vi "Initialize Controls and Indicators.vi"(7 "Set min panel sizes?":bool=TRUE, 8 "error in (no error)":errorcluster, 11 "VI in":refnum<vi>) -> (0 "error out":errorcluster)   [LabVIEW 2020, in "Execution UI V2.lvclass"]
uses:
  Execution UI V2.lvclass
  TypeDefs/Color Theme.ctl
  <vilib>/Utility/miscctls.llb/LVPointTypeDef.ctl
  Execution UI V2.lvclass/Execution UI V2.ctl
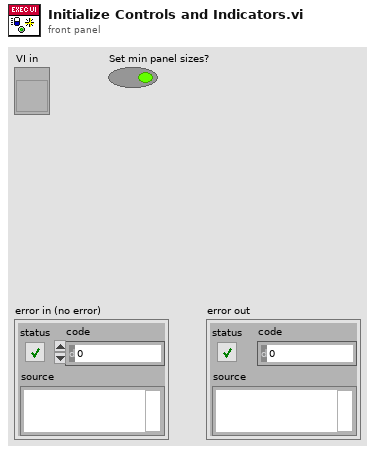
[diagram p1: front panel]
types:
  T1 = typedef "Execution UI V2.lvclass/Color Theme.ctl" = cluster{"Primary":u32, "Primary Light":u32, "Primary Dark":u32, "Accent":u32, "Primary Text":u32, "Secondary Text":u32}
  T2 = typedef "LVPointTypeDef.ctl" = cluster{"Horizontal":i16, "Vertical":i16}
  T3 = enum8{"Enabled", "Disabled", "Disabled and Grayed Out"}
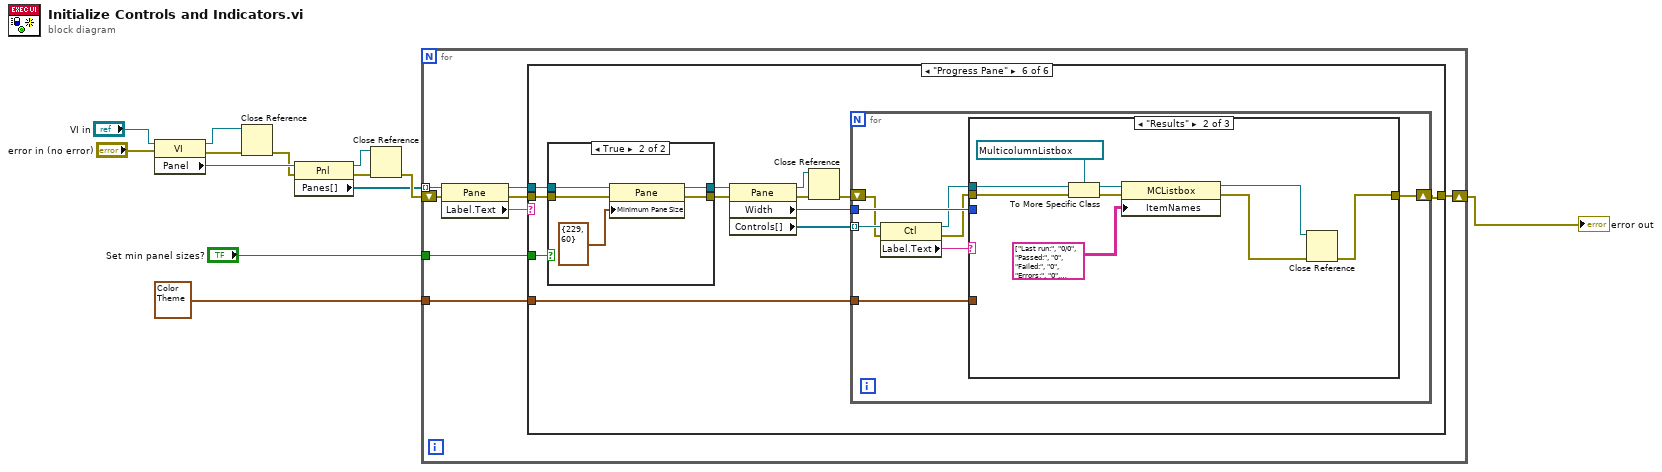
[diagram p0: block diagram]
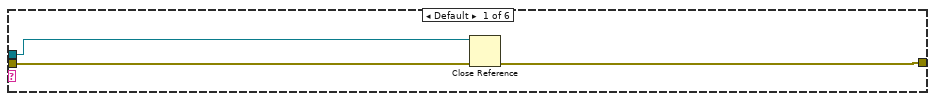
[diagram p2: hidden frame]
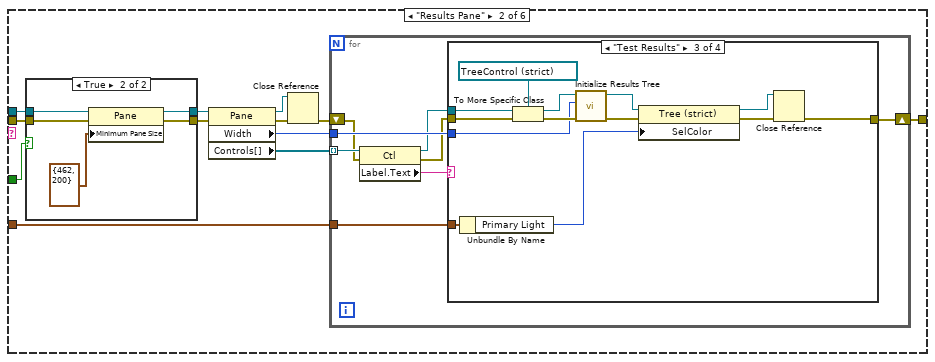
[diagram p3: hidden frame]
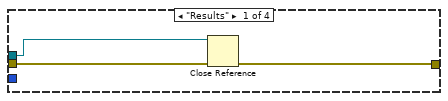
[diagram p5: hidden frame]
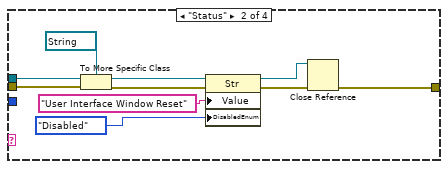
[diagram p6: hidden frame]
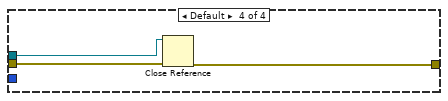
[diagram p7: hidden frame]
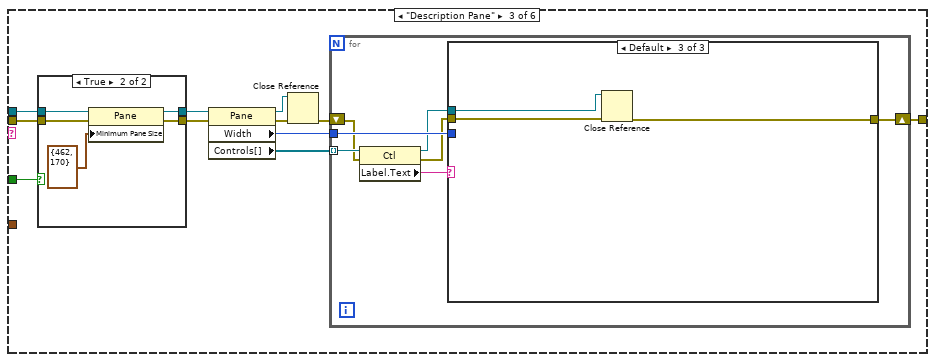
[diagram p8: hidden frame]
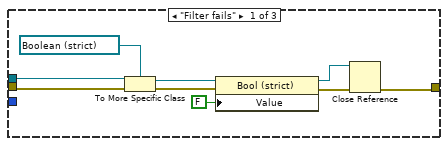
[diagram p10: hidden frame]
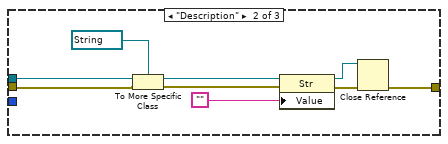
[diagram p11: hidden frame]
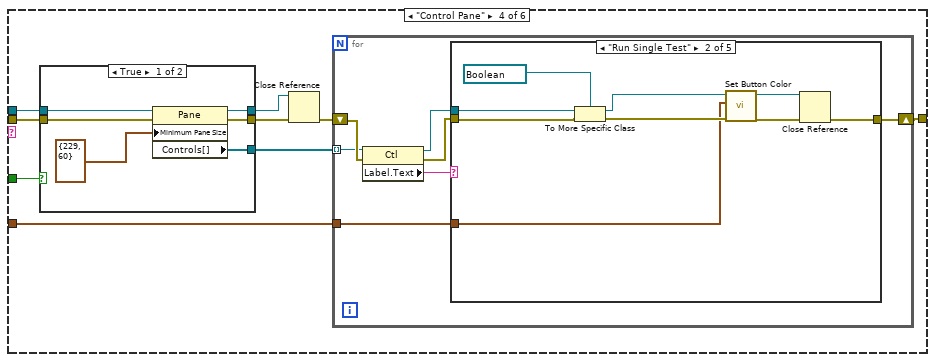
[diagram p12: hidden frame]
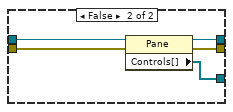
[diagram p13: hidden frame]
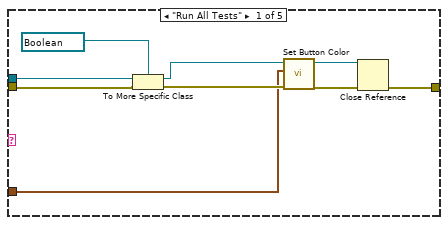
[diagram p14: hidden frame]
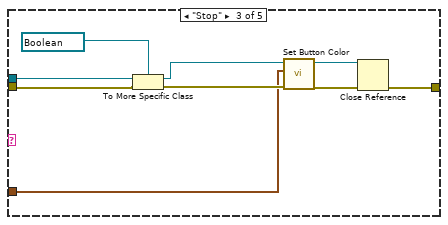
[diagram p15: hidden frame]
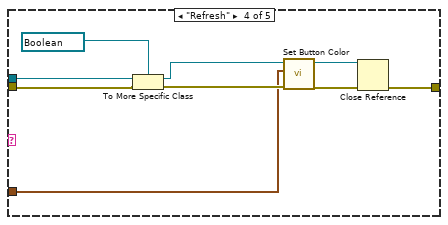
[diagram p16: hidden frame]
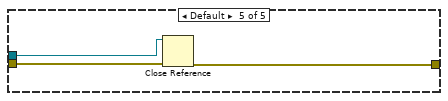
[diagram p17: hidden frame]
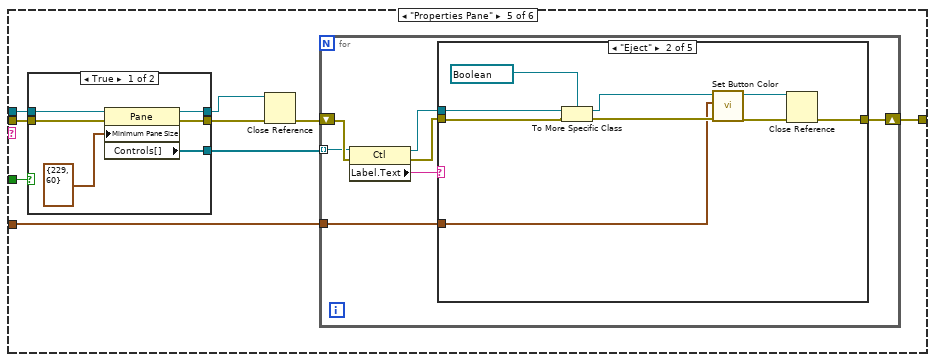
[diagram p18: hidden frame]
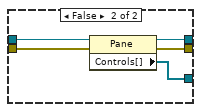
[diagram p19: hidden frame]
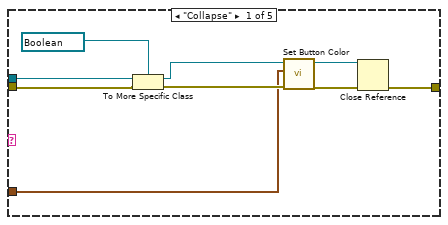
[diagram p20: hidden frame]
diagram:
  n1 = property class="VI"(reference="VI in", error in="error in (no error)") -> (reference out=w3:refnum<vi>, error out=w5:errorcluster, "Panel"=w12:refnum<vi>)
  n2 = Close Reference(reference=w3, error in (no error)=w5) -> (error out=w4:errorcluster)
  n3 = property class="Pnl"(reference=w12, error in=w4) -> (reference out=w8:refnum<vi>, error out=w7:errorcluster, "Panes[]"=w6:refnum<vi>[])
  n4 = Close Reference(reference=w8, error in (no error)=w7) -> (error out=w9:errorcluster)
  n5 = for {
    tunnel: w6 -> [w21] mode=indexing
    shift-right: [w18] -> w10
    shift-left: w9 -> [w17]
    tunnel: T1 {"Primary"=6323595, "Primary Light"=13621468, "Primary Dark"=4545124, "Accent"=10395294, "Primary Text"=2171169, "Secondary Text"=7697781} ("Color Theme") -> [w15]
    tunnel: "Set min panel sizes?" -> [w14]
    n6 = property class="Pane"(reference=w21, error in=w17) -> (reference out=w19:refnum<vi>, error out=w16:errorcluster, "Label.Text"=w20:string)
    n7 = case shown="\"Progress Pane\"" w20 {
      tunnel: w19 -> [w22 w29 w84 w135 w201 w262]
      tunnel: [w23 w34 w89 w130 w196 w261] -> w18
      tunnel: w16 -> [w24 w27 w82 w134 w200 w263]
      tunnel: w15 -> [_ w26 _ w129 w194 w260]
      tunnel: w14 -> [_ w25 w81 w127 w193 w259]
      frame Default {
        n8 = Close Reference(reference=w22, error in (no error)=w24) -> (error out=w23:errorcluster)
      }
      frame "Results Pane" {
        n9 = case shown="True" w25 {
          tunnel: [w38 w43] -> w30
          tunnel: w29 -> [w38 w42]
          tunnel: [w37 w41] -> w28
          tunnel: w27 -> [w37 w40]
          frame False {
          }
          frame True {
            n10 = property class="Pane"(reference=w42, error in=w40, "Minimum Pane Size"=T2 {"Horizontal"=462, "Vertical"=200}) -> (reference out=w43:refnum<vi>, error out=w41:errorcluster)
          }
        }
        n11 = property class="Pane"(reference=w30, error in=w28) -> (reference out=w31:refnum<vi>, error out=w33:errorcluster, "Width"=w36:u32, "Controls[]"=w35:refnum<vi>[])
        n12 = Close Reference(reference=w31, error in (no error)=w33) -> (error out=w32:errorcluster)
        n13 = for {
          tunnel: w36 -> [w51]
          tunnel: w35 -> [w50] mode=indexing
          shift-right: [w45] -> w34
          shift-left: w32 -> [w46]
          tunnel: w26 -> [w44]
          n14 = property class="Ctl"(reference=w50, error in=w46) -> (reference out=w48:refnum<vi>, error out=w47:errorcluster, "Label.Text"=w49:string)
          n15 = case shown="\"Test Results\"" w49 {
            tunnel: w51 -> [_ _ w72 _]
            tunnel: w48 -> [w52 w63 w76 w78]
            tunnel: w47 -> [w54 w62 w77 w80]
            tunnel: [w53 w56 w68 w79] -> w45
            tunnel: w44 -> [_ _ w66 _]
            frame "Results" {
              n16 = Close Reference(reference=w52, error in (no error)=w54) -> (error out=w53:errorcluster)
            }
            frame "Status" {
              n17 = To More Specific Class(target class=refnum<vi> refnum ("reference"), reference=w63, error in=w62) -> (specific class reference=w61:refnum<vi>, error out=w60:errorcluster)
              n18 = property on="Property Node" class="Str"(reference=w61, error in=w60, "Value"="User Interface Window Reset" ("Item Names"), "DisabledEnum"=T3."Disabled" ("Disabled")) -> (reference out=w57:refnum<vi>, error out=w58:errorcluster)
              n19 = Close Reference(reference=w57, error in (no error)=w58) -> (error out=w56:errorcluster)
            }
            frame "Test Results" {
              n20 = Unbundle By Name(w66) -> ("Primary Light"=w65:u32)
              n21 = To More Specific Class(target class=refnum<vi> refnum ("reference"), reference=w76, error in=w77) -> (specific class reference=w74:refnum<vi>, error out=w75:errorcluster)
              n22 = call "Initialize Results Tree.vi"("error in (no error)"=w75, "Pane width"=w72, "TreeControl in"=w74) -> ("error out"=w70:errorcluster, "reference out"=w71:refnum<vi>)  [unwired: 7 in]
              n23 = property class="Tree (strict)"(reference=w71, error in=w70, "SelColor"=w65) -> (reference out=w67:refnum<vi>, error out=w69:errorcluster)
              n24 = Close Reference(reference=w67, error in (no error)=w69) -> (error out=w68:errorcluster)
            }
            frame Default {
              n25 = Close Reference(reference=w78, error in (no error)=w80) -> (error out=w79:errorcluster)
            }
          }
        }
      }
      frame "Description Pane" {
        n26 = case shown="True" w81 {
          tunnel: [w93 w98] -> w85
          tunnel: w84 -> [w93 w97]
          tunnel: [w92 w96] -> w83
          tunnel: w82 -> [w92 w95]
          frame False {
          }
          frame True {
            n27 = property class="Pane"(reference=w97, error in=w95, "Minimum Pane Size"=T2 {"Horizontal"=462, "Vertical"=170}) -> (reference out=w98:refnum<vi>, error out=w96:errorcluster)
          }
        }
        n28 = property class="Pane"(reference=w85, error in=w83) -> (reference out=w86:refnum<vi>, error out=w88:errorcluster, "Width"=w91:u32, "Controls[]"=w90:refnum<vi>[])
        n29 = Close Reference(reference=w86, error in (no error)=w88) -> (error out=w87:errorcluster)
        n30 = for {
          tunnel: w91 -> [w105]
          tunnel: w90 -> [w104] mode=indexing
          shift-right: [w99] -> w89
          shift-left: w87 -> [w100]
          n31 = property class="Ctl"(reference=w104, error in=w100) -> (reference out=w102:refnum<vi>, error out=w101:errorcluster, "Label.Text"=w103:string)
          n32 = case shown="Default" w103 {
            tunnel: w105 -> [_ _ _]
            tunnel: w102 -> [w108 w123 w124]
            tunnel: w101 -> [w109 w118 w126]
            tunnel: [w110 w120 w125] -> w99
            frame "Filter fails" {
              n33 = To More Specific Class(target class=refnum<vi> refnum ("Filter fails"), reference=w108, error in=w109) -> (specific class reference=w112:refnum<vi>, error out=w111:errorcluster)
              n34 = property on="Property Node" class="Bool (strict)"(reference=w112, error in=w111, "Value"=FALSE) -> (reference out=w113:refnum<vi>, error out=w114:errorcluster)
              n35 = Close Reference(reference=w113, error in (no error)=w114) -> (error out=w110:errorcluster)
            }
            frame "Description" {
              n36 = To More Specific Class(target class=refnum<vi> refnum ("reference"), reference=w123, error in=w118) -> (specific class reference=w119:refnum<vi>, error out=w117:errorcluster)
              n37 = property on="Property Node" class="Str"(reference=w119, error in=w117, "Value"="") -> (reference out=w121:refnum<vi>, error out=w122:errorcluster)
              n38 = Close Reference(reference=w121, error in (no error)=w122) -> (error out=w120:errorcluster)
            }
            frame Default {
              n39 = Close Reference(reference=w124, error in (no error)=w126) -> (error out=w125:errorcluster)
            }
          }
        }
      }
      frame "Control Pane" {
        n40 = case shown="True" w127 {
          tunnel: w135 -> [w140 w146]
          tunnel: w134 -> [w139 w145]
          tunnel: [w138 w144] -> w133
          tunnel: [w137 w143] -> w132
          tunnel: [w136 w142] -> w128
          frame True {
            n41 = property class="Pane"(reference=w140, error in=w139, "Minimum Pane Size"=T2 {"Horizontal"=229, "Vertical"=60}) -> (reference out=w137:refnum<vi>, error out=w138:errorcluster, "Controls[]"=w136:refnum<vi>[])
          }
          frame False {
            n42 = property class="Pane"(reference=w146, error in=w145) -> (reference out=w143:refnum<vi>, error out=w144:errorcluster, "Controls[]"=w142:refnum<vi>[])
          }
        }
        n43 = Close Reference(reference=w132, error in (no error)=w133) -> (error out=w131:errorcluster)
        n44 = for {
          shift-right: [w149] -> w130
          shift-left: w131 -> [w150]
          tunnel: w129 -> [w148]
          tunnel: w128 -> [w147] mode=indexing
          n45 = property class="Ctl"(reference=w147, error in=w150) -> (reference out=w152:refnum<vi>, error out=w151:errorcluster, "Label.Text"=w153:string)
          n46 = case shown="\"Run Single Test\"" w153 {
            tunnel: w152 -> [w162 w171 w180 w189 w190]
            tunnel: w151 -> [w160 w169 w178 w187 w192]
            tunnel: [w161 w170 w179 w188 w191] -> w149
            tunnel: w148 -> [w154 w163 w172 w181 _]
            frame "Run All Tests" {
              n47 = To More Specific Class(target class=refnum<vi> refnum ("Status"), reference=w162, error in=w160) -> (specific class reference=w158:refnum<vi>, error out=w157:errorcluster)
              n48 = call "Set Button Color.vi"("error in (no error)"=w157, "Color Theme"=w154, "Reference in"=w158) -> ("error out"=w155:errorcluster, "Reference out"=w156:refnum<vi>)  [unwired: 7 in]
              n49 = Close Reference(reference=w156, error in (no error)=w155) -> (error out=w161:errorcluster)
            }
            frame "Run Single Test" {
              n50 = To More Specific Class(target class=refnum<vi> refnum ("Status"), reference=w171, error in=w169) -> (specific class reference=w167:refnum<vi>, error out=w166:errorcluster)
              n51 = call "Set Button Color.vi"("error in (no error)"=w166, "Color Theme"=w163, "Reference in"=w167) -> ("error out"=w164:errorcluster, "Reference out"=w165:refnum<vi>)  [unwired: 7 in]
              n52 = Close Reference(reference=w165, error in (no error)=w164) -> (error out=w170:errorcluster)
            }
            frame "Stop" {
              n53 = To More Specific Class(target class=refnum<vi> refnum ("Status"), reference=w180, error in=w178) -> (specific class reference=w176:refnum<vi>, error out=w175:errorcluster)
              n54 = call "Set Button Color.vi"("error in (no error)"=w175, "Color Theme"=w172, "Reference in"=w176) -> ("error out"=w173:errorcluster, "Reference out"=w174:refnum<vi>)  [unwired: 7 in]
              n55 = Close Reference(reference=w174, error in (no error)=w173) -> (error out=w179:errorcluster)
            }
            frame "Refresh" {
              n56 = To More Specific Class(target class=refnum<vi> refnum ("Status"), reference=w189, error in=w187) -> (specific class reference=w185:refnum<vi>, error out=w184:errorcluster)
              n57 = call "Set Button Color.vi"("error in (no error)"=w184, "Color Theme"=w181, "Reference in"=w185) -> ("error out"=w182:errorcluster, "Reference out"=w183:refnum<vi>)  [unwired: 7 in]
              n58 = Close Reference(reference=w183, error in (no error)=w182) -> (error out=w188:errorcluster)
            }
            frame Default {
              n59 = Close Reference(reference=w190, error in (no error)=w192) -> (error out=w191:errorcluster)
            }
          }
        }
      }
      frame "Properties Pane" {
        n60 = case shown="True" w193 {
          tunnel: w201 -> [w206 w212]
          tunnel: w200 -> [w205 w211]
          tunnel: [w204 w210] -> w199
          tunnel: [w203 w209] -> w198
          tunnel: [w202 w208] -> w195
          frame True {
            n61 = property class="Pane"(reference=w206, error in=w205, "Minimum Pane Size"=T2 {"Horizontal"=229, "Vertical"=60}) -> (reference out=w203:refnum<vi>, error out=w204:errorcluster, "Controls[]"=w202:refnum<vi>[])
          }
          frame False {
            n62 = property class="Pane"(reference=w212, error in=w211) -> (reference out=w209:refnum<vi>, error out=w210:errorcluster, "Controls[]"=w208:refnum<vi>[])
          }
        }
        n63 = Close Reference(reference=w198, error in (no error)=w199) -> (error out=w197:errorcluster)
        n64 = for {
          shift-right: [w215] -> w196
          shift-left: w197 -> [w216]
          tunnel: w194 -> [w214]
          tunnel: w195 -> [w213] mode=indexing
          n65 = property class="Ctl"(reference=w213, error in=w216) -> (reference out=w218:refnum<vi>, error out=w217:errorcluster, "Label.Text"=w219:string)
          n66 = case shown="\"Eject\"" w219 {
            tunnel: w218 -> [w228 w237 w246 w255 w256]
            tunnel: w217 -> [w226 w235 w244 w253 w258]
            tunnel: [w227 w236 w245 w254 w257] -> w215
            tunnel: w214 -> [w220 w229 w238 w247 _]
            frame "Collapse" {
              n67 = To More Specific Class(target class=refnum<vi> refnum ("Status"), reference=w228, error in=w226) -> (specific class reference=w224:refnum<vi>, error out=w223:errorcluster)
              n68 = call "Set Button Color.vi"("error in (no error)"=w223, "Color Theme"=w220, "Reference in"=w224) -> ("error out"=w221:errorcluster, "Reference out"=w222:refnum<vi>)  [unwired: 7 in]
              n69 = Close Reference(reference=w222, error in (no error)=w221) -> (error out=w227:errorcluster)
            }
            frame "Eject" {
              n70 = To More Specific Class(target class=refnum<vi> refnum ("Status"), reference=w237, error in=w235) -> (specific class reference=w233:refnum<vi>, error out=w232:errorcluster)
              n71 = call "Set Button Color.vi"("error in (no error)"=w232, "Color Theme"=w229, "Reference in"=w233) -> ("error out"=w230:errorcluster, "Reference out"=w231:refnum<vi>)  [unwired: 7 in]
              n72 = Close Reference(reference=w231, error in (no error)=w230) -> (error out=w236:errorcluster)
            }
            frame "Expand" {
              n73 = To More Specific Class(target class=refnum<vi> refnum ("Status"), reference=w246, error in=w244) -> (specific class reference=w242:refnum<vi>, error out=w241:errorcluster)
              n74 = call "Set Button Color.vi"("error in (no error)"=w241, "Color Theme"=w238, "Reference in"=w242) -> ("error out"=w239:errorcluster, "Reference out"=w240:refnum<vi>)  [unwired: 7 in]
              n75 = Close Reference(reference=w240, error in (no error)=w239) -> (error out=w245:errorcluster)
            }
            frame "Save" {
              n76 = To More Specific Class(target class=refnum<vi> refnum ("Status"), reference=w255, error in=w253) -> (specific class reference=w251:refnum<vi>, error out=w250:errorcluster)
              n77 = call "Set Button Color.vi"("error in (no error)"=w250, "Color Theme"=w247, "Reference in"=w251) -> ("error out"=w248:errorcluster, "Reference out"=w249:refnum<vi>)  [unwired: 7 in]
              n78 = Close Reference(reference=w249, error in (no error)=w248) -> (error out=w254:errorcluster)
            }
            frame Default {
              n79 = Close Reference(reference=w256, error in (no error)=w258) -> (error out=w257:errorcluster)
            }
          }
        }
      }
      frame "Progress Pane" {
        n80 = case shown="True" w259 {
          tunnel: [w272 w277] -> w265
          tunnel: [w271 w276] -> w264
          tunnel: w263 -> [w271 w275]
          tunnel: w262 -> [w272 w274]
          frame False {
          }
          frame True {
            n81 = property class="Pane"(reference=w274, error in=w275, "Minimum Pane Size"=T2 {"Horizontal"=229, "Vertical"=60}) -> (reference out=w277:refnum<vi>, error out=w276:errorcluster)
          }
        }
        n82 = property class="Pane"(reference=w265, error in=w264) -> (reference out=w266:refnum<vi>, error out=w268:errorcluster, "Width"=w270:u32, "Controls[]"=w269:refnum<vi>[])
        n83 = Close Reference(reference=w266, error in (no error)=w268) -> (error out=w267:errorcluster)
        n84 = for {
          tunnel: w270 -> [w285]
          tunnel: w269 -> [w284] mode=indexing
          shift-right: [w279] -> w261
          shift-left: w267 -> [w280]
          tunnel: w260 -> [w278]
          n85 = property class="Ctl"(reference=w284, error in=w280) -> (reference out=w282:refnum<vi>, error out=w281:errorcluster, "Label.Text"=w283:string)
          n86 = case shown="\"Results\"" w283 {
            tunnel: w285 -> [_ _ _]
            tunnel: w282 -> [w292 w302 w307]
            tunnel: w281 -> [w290 w304 w309]
            tunnel: [w294 w306 w308] -> w279
            tunnel: w278 -> [w287 _ _]
            frame "Progress bar" {
              n87 = Unbundle By Name(w287) -> ("Primary"=w286:u32)
              n88 = To More Specific Class(target class=refnum<vi> refnum ("Progress bar"), reference=w292, error in=w290) -> (specific class reference=w291:refnum<vi>, error out=w289:errorcluster)
              n89 = To Variant(anything=0.0 ("Progress bar")) -> (Variant=w293:variant)
              n90 = property on="Property Node" class="Slide"(reference=w291, error in=w289, "Value"=w293, "Fill Color"=w286) -> (reference out=w295:refnum<vi>, error out=w296:errorcluster)
              n91 = Close Reference(reference=w295, error in (no error)=w296) -> (error out=w294:errorcluster)
            }
            frame "Results" {
              n92 = To More Specific Class(target class=refnum<vi> refnum ("Results"), reference=w302, error in=w304) -> (specific class reference=w300:refnum<vi>, error out=w305:errorcluster)
              n93 = property class="MCListbox"(reference=w300, error in=w305, "ItemNames"=string[][] [["Last run:", "0/0", "Passed:", "0", "Failed:", "0", "Errors:", "0", "Skipped:", "0"]] ("Item Names")) -> (reference out=w299:refnum<vi>, error out=w301:errorcluster)
              n94 = Close Reference(reference=w299, error in (no error)=w301) -> (error out=w306:errorcluster)
            }
            frame Default {
              n95 = Close Reference(reference=w307, error in (no error)=w309) -> (error out=w308:errorcluster)
            }
          }
        }
      }
    }
  }
  "error out" <- w10
